vi "Load Evaluations From File.vi"(8 "error in (no error)":errorcluster, 10 "all rows":string[][](array[string]), 11 "Limit Dictionary in":variant) -> (0 "error out":errorcluster, 3 "Limit Dictionary out":variant)   [LabVIEW 2018, in "Test Number and Bin Generator.lvlib" / "Test Number and Bin Generator.lvclass"]
uses:
  Test Number and Bin Generator.lvclass
  Plugins/TestStand API Tools (TSAT).lvlibp/Evaluation Actions/Includes/Controls/TSAT Evaluation.ctl
  Plugins/TestStand API Tools (TSAT).lvlibp/Evaluation Actions/Includes/Controls/TSAT Eval SI Unit Scaling.ctl
  Plugins/TestStand API Tools (TSAT).lvlibp/Evaluation Actions/Includes/Controls/TSAT Evaluation Type.ctl
  Plugins/TestStand API Tools (TSAT).lvlibp/Evaluation Actions/TSAT Evaluation Actions.lvlib
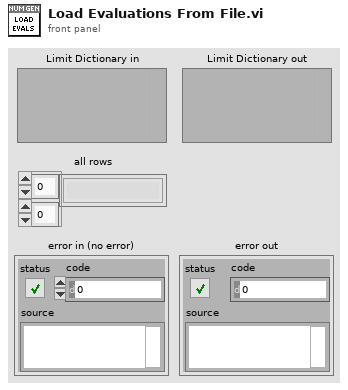
[diagram p1: front panel]
types:
  T1 = typedef "TestStand API Tools (TSAT).lvlibp/TSAT Evaluation Actions.lvlib/TSAT Evaluation.ctl" = cluster{"Test Name":string, "Pin":string, "Units":string, "SI Scaling":T2, "Test Number":i32, "Published Data Id":string, "Low Limit":dbl, "High Limit":dbl, "Export Data Location":string, "Software Bin":i64, "Evaluation Type":T3, "Test Data Source":string}
  T2 = typedef "TestStand API Tools (TSAT).lvlibp/TSAT Evaluation Actions.lvlib/TSAT Eval SI Unit Scaling.ctl" = i16
  T3 = typedef "TestStand API Tools (TSAT).lvlibp/TSAT Evaluation Actions.lvlib/TSAT Evaluation Type.ctl" = enum16{"Numeric Limit", "Pass/Fail", "None"}
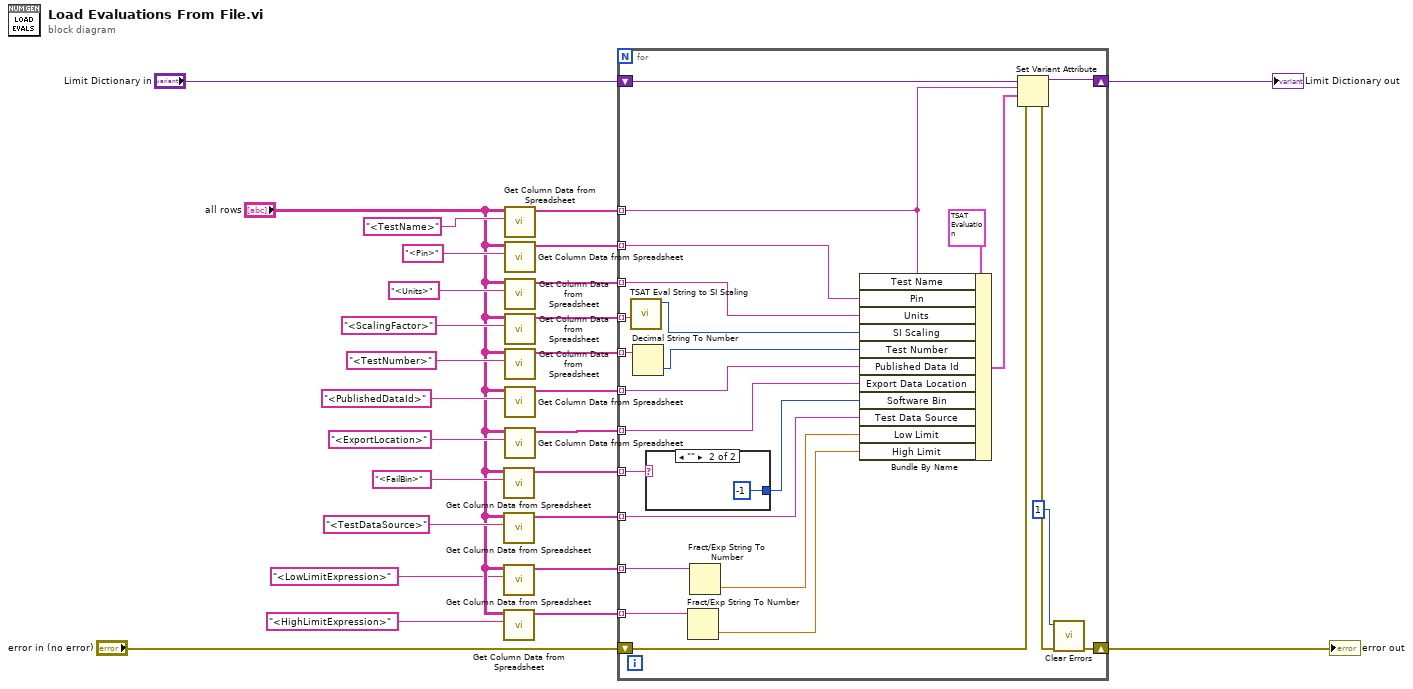
[diagram p0: block diagram]
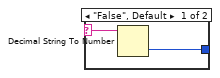
[diagram p2: hidden frame]
diagram:
  n1 = call "Get Column Data from Spreadsheet.vi"("Column Tag"="<FailBin>", "SpreadSheet Data In"="all rows") -> ("Column Data"=w23:string[])  [unwired: 9 in]
  n2 = call "Get Column Data from Spreadsheet.vi"("Column Tag"="<TestDataSource>", "SpreadSheet Data In"="all rows") -> ("Column Data"=w7:string[])  [unwired: 9 in]
  n3 = call "Get Column Data from Spreadsheet.vi"("Column Tag"="<LowLimitExpression>", "SpreadSheet Data In"="all rows") -> ("Column Data"=w2:string[])  [unwired: 9 in]
  n4 = call "Get Column Data from Spreadsheet.vi"("Column Tag"="<HighLimitExpression>", "SpreadSheet Data In"="all rows") -> ("Column Data"=w1:string[])  [unwired: 9 in]
  n5 = call "Get Column Data from Spreadsheet.vi"("Column Tag"="<TestName>", "SpreadSheet Data In"="all rows") -> ("Column Data"=w12:string[])  [unwired: 9 in]
  n6 = call "Get Column Data from Spreadsheet.vi"("Column Tag"="<Pin>", "SpreadSheet Data In"="all rows") -> ("Column Data"=w13:string[])  [unwired: 9 in]
  n7 = call "Get Column Data from Spreadsheet.vi"("Column Tag"="<Units>", "SpreadSheet Data In"="all rows") -> ("Column Data"=w14:string[])  [unwired: 9 in]
  n8 = call "Get Column Data from Spreadsheet.vi"("Column Tag"="<ScalingFactor>", "SpreadSheet Data In"="all rows") -> ("Column Data"=w15:string[])  [unwired: 9 in]
  n9 = call "Get Column Data from Spreadsheet.vi"("Column Tag"="<TestNumber>", "SpreadSheet Data In"="all rows") -> ("Column Data"=w17:string[])  [unwired: 9 in]
  n10 = call "Get Column Data from Spreadsheet.vi"("Column Tag"="<PublishedDataId>", "SpreadSheet Data In"="all rows") -> ("Column Data"=w19:string[])  [unwired: 9 in]
  n11 = call "Get Column Data from Spreadsheet.vi"("Column Tag"="<ExportLocation>", "SpreadSheet Data In"="all rows") -> ("Column Data"=w21:string[])  [unwired: 9 in]
  n12 = for {
    tunnel: w12 -> [w38] mode=indexing
    tunnel: w13 -> [w50] mode=indexing
    tunnel: w14 -> [w49] mode=indexing
    tunnel: w15 -> [w48] mode=indexing
    tunnel: w17 -> [w46] mode=indexing
    tunnel: w19 -> [w44] mode=indexing
    tunnel: w21 -> [w43] mode=indexing
    tunnel: w23 -> [w42] mode=indexing
    shift-right: [w39] -> w25
    shift-left: "Limit Dictionary in" -> [w40]
    shift-right: [w34] -> w27
    shift-left: "error in (no error)" -> [w36]
    tunnel: w7 -> [w32] mode=indexing
    tunnel: w2 -> [w31] mode=indexing
    tunnel: w1 -> [w30] mode=indexing
    n13 = call "TSAT Eval String to SI Scaling.vi"("String"=w48) -> ("SI Scaling"=w47:T2)  [unwired: 10 in]
    n14 = Decimal String To Number(string=w46) -> (number=w45:i32)  [unwired: 2 in, 1 out]
    n15 = case shown="\"\"" w42 {
      selector: w42 -> [w53 _]
      tunnel: [w52 -1] -> w41
      frame "False", Default {
        n16 = Decimal String To Number(string=w53) -> (number=w52:i32)  [unwired: 2 in, 1 out]
      }
      frame "" {
      }
    }
    n17 = Fract/Exp String To Number(string=w30) -> (number=w28:dbl)  [unwired: 3 in, 1 out]
    n18 = Fract/Exp String To Number(string=w31) -> (number=w29:dbl)  [unwired: 3 in, 1 out]
    n19 = Bundle By Name(cluster=T1 {"Test Name"="", "Pin"="", "Units"="", "SI Scaling"=0, "Test Number"=0, "Published Data Id"="", "Low Limit"=0.0, "High Limit"=0.0, "Export Data Location"="", "Software Bin"=0, "Evaluation Type"=enum."Numeric Limit", "Test Data Source"=""} ("Evaluation"), "Test Name"=w38, "Pin"=w50, "Units"=w49, "SI Scaling"=w47, "Test Number"=w45, "Published Data Id"=w44, "Export Data Location"=w43, "Software Bin"=w41, "Test Data Source"=w32, "Low Limit"=w29, "High Limit"=w28) -> (w37:T1)
    n20 = Set Variant Attribute(Variant=w40, name=w38, value=w37, error in=w36) -> (Variant out=w39:variant, error out=w35:errorcluster)  [unwired: 1 out]
    n21 = call <vilib>:"Clear Errors.vi"("error in (no error)"=w35, "specific error code to clear (0: all)"=1) -> ("error out"=w34:errorcluster)  [unwired: 4 in, 1 out]
  }
  "error out" <- w27
  "Limit Dictionary out" <- w25
